vi "_DEPRICATED FRCts20_WebMethods_Team_POST.vi"(7 "httpRequestID":u32) -> ()   [LabVIEW 2014, in "FRCts20_WebMethods.lvlib"]
doc: "<B>POST</B> a new team resource\n\n<B>Required XML Data : </B>\n<Team>\n <TeamNumber><B>uInt</B></TeamNumber>\n <SWType>[<B>unknown</B>, <B>LabVIEW</B>, <B>Windriver, C++</B>, <B>JavaBeans</B>, <B>Other</B>]</SWType>\n <Division><B>string</B></Division>\n</Team>\n\nhttp://<server address>:<port>/FRCts/team\n\n{requires authentication}"
uses:
  FRCts20_WebMethods.lvlib
  Backend/source/VI Source/FRCts20_Backend_API/FRCts20_Backend_API_Team.ctl
  Backend/source/VI Source/FRCts20_Backend_API/FRCts20_Backend_API.lvlib
  <vilib>/wsapi/NI_WebServices.lvlib
  Backend/source/VI Source/FRCts20_Backend_API/FRCts20_Backend_API_Command_Team.ctl
  Backend/source/VI Source/FRCts20_Backend_API/FRCts20_Backend_API_TeamRoot.ctl
  Backend/source/VI Source/FRCts20_Backend_API/FRCts20_Backend_API_TeamRoot.vi
  FRCts20_WebMethods_ReadData_Team.vi
  Backend/source/VI Source/FRCts20_Backend_API/FRCts20_Backend_API_Team.vi
  Backend/source/VI Source/FRCts20_Backend_API/FRCts20_Backend_API_Status.ctl
  Backend/source/VI Source/FRCts20_Backend_API/FRCts20_Backend_API_SW.ctl
  FRCts20_WebMethods_Redirect_Request.vi
panel:
  in  "query":string
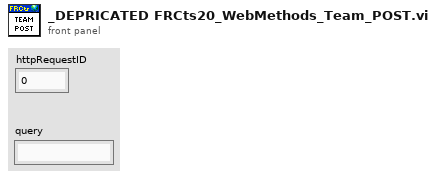
[diagram p1: front panel]
types:
  T1 = typedef "FRCts20_Backend_Engine.lvlib/FRCts20_Backend_API.lvlib/FRCts20_Backend_API_Team.ctl" = cluster{"Team Index":u32, "Team Number":u32, "Team Name":string, "Short Team Name":string, "Nick Name":string, "Robot Name":string, "City":string, "State":string, "Country":string, "Rookie Year":u32, "SWType":T2, "CAN":bool, "Vision":bool, "Kinect":bool, "Tags":string, "Avatar":string, "Request Array":cluster{"Request Index":u32, "Description":string, "Status":T3, "Open Date":timestamp, "Last Update":timestamp, "Close Date":timestamp}[], "Events Attending":cluster{"EventIndex":i32, "EventName":string, "IsLive":bool}[], "APIReturn":string}
  T2 = typedef "FRCts20_Backend_Engine.lvlib/FRCts20_Backend_API.lvlib/FRCts20_Backend_API_SW.ctl" = string
  T3 = typedef "FRCts20_Backend_Engine.lvlib/FRCts20_Backend_API.lvlib/FRCts20_Backend_API_Status.ctl" = i32
  T4 = typedef "FRCts20_Backend_API.lvlib/FRCts20_Backend_API_Command_TeamRoot.ctl" = string
  T5 = typedef "FRCts20_Backend_Engine.lvlib/FRCts20_Backend_API.lvlib/FRCts20_Backend_API_Command_Team.ctl" = string
  T6 = typedef "FRCts20_Backend_Engine.lvlib/FRCts20_Backend_API.lvlib/FRCts20_Backend_API_TeamRoot.ctl" = cluster{"Teams":cluster{"Team Index":u32, "Team Number":u32, "Team ID":u32, "Team Name":string, "Short Team Name":string, "Nick Name":string, "Robot Name":string, "City":string, "State":string, "Country":string, "Rookie Year":u32, "SWType":T2, "CAN":bool, "Vision":bool, "Kinect":bool, "Tags":string, "Avatar":string, "Events":cluster{"EventIndex":u32, "EventName":string, "IsLive":bool}[]}[], "APIReturn":string}
  T7 = typedef "FRCts20_Backend_Engine.lvlib/FRCts20_Backend_API.lvlib/Team.ctl" = cluster{"APIReturn":T8, "TeamRoot":T9, "TeamExtendedData":T10, "Events":T11[]}
  T8 = typedef "FRCts20_Backend_Engine.lvlib/FRCts20_Backend_API.lvlib/ApiReturn.ctl" = string
  T9 = typedef "FRCts20_Backend_Engine.lvlib/FRCts20_Backend_API.lvlib/TeamRoot.ctl" = cluster{"TeamIndex":i32, "TeamNumber":u32, "SoftwareType":T2}
  T10 = typedef "FRCts20_Backend_Engine.lvlib/FRCts20_Backend_API.lvlib/TeamExtended.ctl" = cluster{"TeamName":string, "ShortTeamName":string, "NickName":string, "RobotName":string, "City":string, "State":string, "Country":string, "RookieYear":u32, "CAN":bool, "Vision":bool, "Kinect":bool, "Avatar":string, "Team ID":u32, "Tags":string}
  T11 = typedef "FRCts20_Backend_Engine.lvlib/FRCts20_Backend_API.lvlib/EventRoot.ctl" = cluster{"EventIndex":i32, "EventName":string, "IsLive":bool, "OpenIssues":i32}
  T12 = cluster{"Team Index":u32, "Team Number":u32, "Team ID":u32, "Team Name":string, "Short Team Name":string, "Nick Name":string, "Robot Name":string, "City":string, "State":string, "Country":string, "Rookie Year":u32, "SWType":T2, "CAN":bool, "Vision":bool, "Kinect":bool, "Tags":string, "Avatar":string, "Events":cluster{"EventIndex":u32, "EventName":string, "IsLive":bool}[]}[]
  T13 = cluster{"Team Index":u32, "Team Number":u32, "Team ID":u32, "Team Name":string, "Short Team Name":string, "Nick Name":string, "Robot Name":string, "City":string, "State":string, "Country":string, "Rookie Year":u32, "SWType":T2, "CAN":bool, "Vision":bool, "Kinect":bool, "Tags":string, "Avatar":string, "Events":cluster{"EventIndex":u32, "EventName":string, "IsLive":bool}[]}
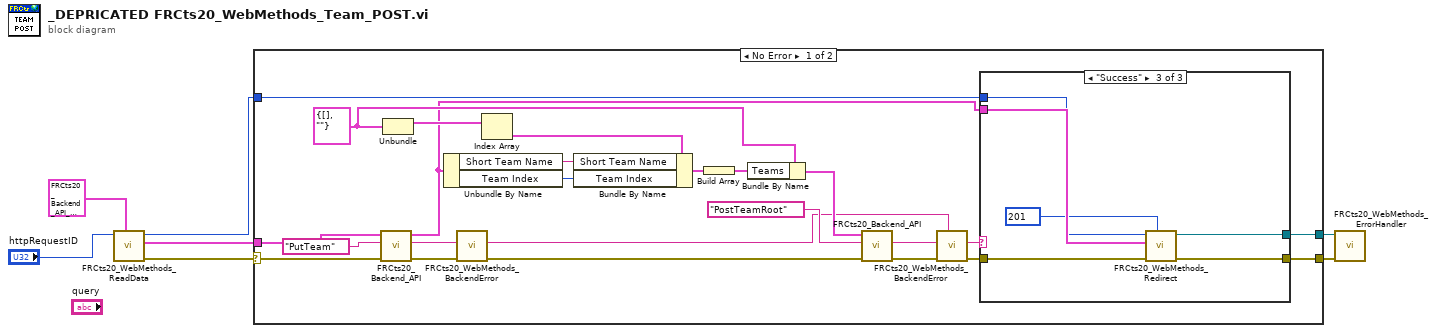
[diagram p0: block diagram]
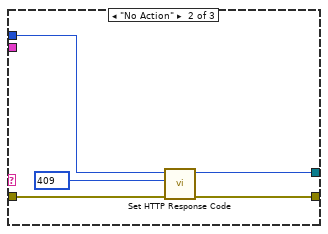
[diagram p3: hidden frame]
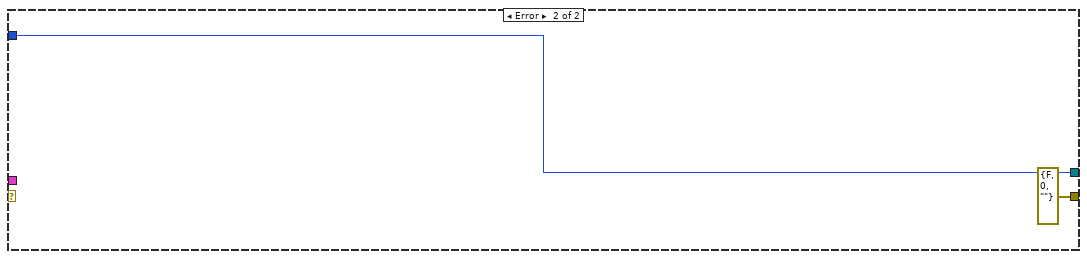
[diagram p4: hidden frame]
diagram:
  n1 = call-poly "FRCts20_WebMethods_ReadData.vi"("Team"=T1 {"Team Index"=0, "Team Number"=0, "Team Name"="", "Short Team Name"="", "Nick Name"="", "Robot Name"="", "City"="", "State"="", "Country"="", "Rookie Year"=0, "SWType"="", "CAN"=FALSE, "Vision"=FALSE, "Kinect"=FALSE, "Tags"="", "Avatar"="", "Request Array"=[], "Events Attending"=[], "APIReturn"=""}, "httpRequestID"="httpRequestID") -> ("error out"=w3:errorcluster, "Team Out"=w4:T1, "httpRequestID out"=w1:u32)  [unwired: 7 in]
  n2 = case shown="No Error" w3 {
    selector: w3 -> [w8 _]
    tunnel: [w31 errorcluster {"status"=FALSE, "code"=0, "source"=""} ("error out")] -> w6
    tunnel: [w30 w46] -> w5
    tunnel: w1 -> [w27 w46]
    tunnel: w4 -> [w26 _]
    frame No Error {
      w15 = T6 {"Teams"=[], "APIReturn"=""} ("Team In")
      n3 = call-poly "FRCts20_Backend_API.vi"("error in (no error)"=w8, "Command"=T5 "PutTeam", "Team In"=w26) -> ("error out"=w29:errorcluster, "Status"=w28:string, "Team Out"=w11:T7)  [unwired: 6 in]
      n4 = Unbundle(w15) -> ("Teams"=w14:T12)  [unwired: 1 out]
      n5 = Unbundle By Name(w11) -> ("Short Team Name"=w18:string, "Team Index"=w10:u32)
      n6 = call "FRCts20_WebMethods_BackendError.vi"("error in (no error)"=w29, "Status"=w28) -> ("error out"=w12:errorcluster, "Status out"=w9:string)  [unwired: 8 in]
      n7 = Index Array(array=w14) -> (element=w13:T13)  [unwired: 1 in]
      n8 = Bundle By Name(cluster=w13, "Short Team Name"=w18, "Team Index"=w10) -> (w17:T13)
      n9 = Build Array(w17) -> (w16:T12)
      n10 = Bundle By Name(cluster=w15, "Teams"=w16) -> (w19:T6)
      n11 = call-poly "FRCts20_Backend_API.vi"("error in (no error)"=w12, "Command"=T4 "PostTeamRoot", "Teams In"=w19) -> ("error out"=w24:errorcluster, "Status"=w23:string)  [unwired: 6 in, 1 out]
      n12 = call "FRCts20_WebMethods_BackendError.vi"("Prev Status"=w9, "error in (no error)"=w24, "Status"=w23) -> ("error out"=w21:errorcluster, "Status out"=w22:string)  [unwired: 7 in]
      n13 = case shown="\"Success\"" w22 {
        tunnel: [w33 w38 w44] -> w31
        tunnel: [w32 w37 w43] -> w30
        tunnel: w11 -> [_ _ w42]
        tunnel: w21 -> [w33 w36 w41]
        tunnel: w27 -> [w32 w35 w40]
        frame "Backend Error", Default {
        }
        frame "No Action" {
          w34 = 409 items=["100"=100, "101"=101, "200"=200, "201"=201, "202"=202, "203"=203, "204"=204, "205"=205, "206"=206, "300"=300, "301"=301, "302"=302, "303"=303, "304"=304, "305"=305, "306"=306, "307"=307, "400"=400, "401"=401, "402"=402, "403"=403, "404"=404, "405"=405, "406"=406, "407"=407, "408"=408, "409"=409, "410"=410, "411"=411, "412"=412, "413"=413, "414"=414, "415"=415, "416"=416, "417"=417, "500"=500, "501"=501, "502"=502, "503"=503, "504"=504, "505"=505] ("response code (200)")
          n14 = call <vilib>:"Set HTTP Response Code.vi"("error in (no error)"=w36, "response code (200)"=w34, "httpRequestID"=w35) -> ("error out"=w38:errorcluster, "httpRequestID out"=w37:u32)  [unwired: 7 in]
        }
        frame "Success" {
          w39 = 201 items=["100"=100, "101"=101, "200"=200, "201"=201, "202"=202, "203"=203, "204"=204, "205"=205, "206"=206, "300"=300, "301"=301, "302"=302, "303"=303, "304"=304, "305"=305, "306"=306, "307"=307, "400"=400, "401"=401, "402"=402, "403"=403, "404"=404, "405"=405, "406"=406, "407"=407, "408"=408, "409"=409, "410"=410, "411"=411, "412"=412, "413"=413, "414"=414, "415"=415, "416"=416, "417"=417, "500"=500, "501"=501, "502"=502, "503"=503, "504"=504, "505"=505] ("response code (200)")
          n15 = call-poly "FRCts20_WebMethods_Redirect.vi"("response code (307)"=w39, "error in (no error)"=w41, "Request"=w42, "LabVIEW Web Service Request"=w40) -> ("error out"=w44:errorcluster, "LabVIEW Web Service Request out"=w43:refnum<class "Web Request.lvclass">)  [unwired: 6 in]
        }
      }
    }
    frame Error {
    }
  }
  n16 = call "FRCts20_WebMethods_ErrorHandler.vi"("error in"=w6, "LabVIEW Web Service Request"=w5) -> ()  [unwired: 8 in, 2 out]
